vi "getValue.vi"(8 "error in (no error)":errorcluster, 11 "tBSONArray in":refnum<class "tBSONArray.lvclass">) -> (0 "error out":errorcluster, 2 "Value":refnum<class "tBSONElement.lvclass">[](array[class]), 3 "tBSONArray out":refnum<class "tBSONArray.lvclass">)   [LabVIEW 2013, in "BSON.lvlib" / "tBSONArray.lvclass"]
uses:
  tBSONArray.lvclass
  tBSONElement/tBSONElement.lvclass
  tBSONArray.lvclass/tBSONArray.ctl
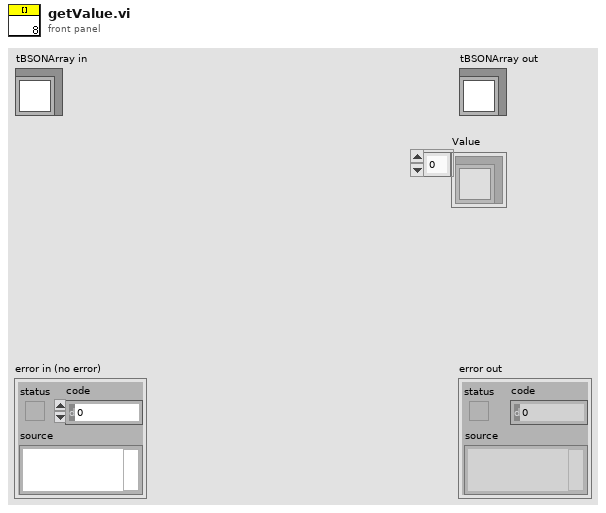
[diagram p1: front panel]
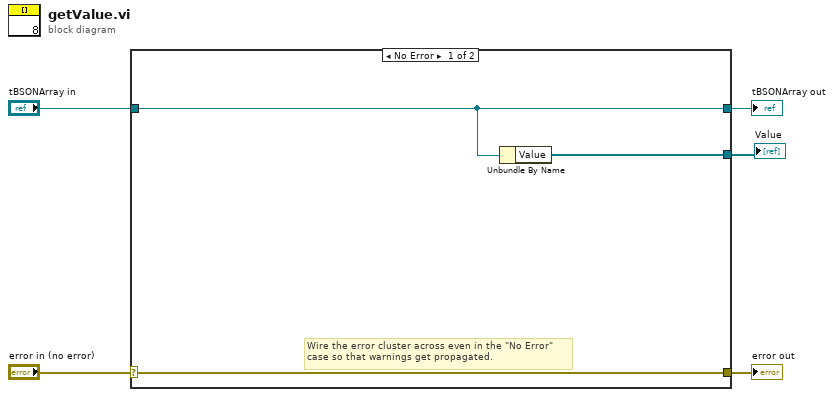
[diagram p0: block diagram]
diagram:
  n1 = case shown="No Error" "error in (no error)" {
    selector: "error in (no error)" -> [w8 w10]
    tunnel: [w8 w10] -> w4
    tunnel: [w7 w9] -> w2
    tunnel: "tBSONArray in" -> [w7 w9]
    tunnel: [w6 _] -> w1
    frame No Error {
      # "Wire the error cluster across even in the \"No Error\"\ncase so that warnings get propagated."
      n2 = Unbundle By Name(w7) -> ("Value"=w6:refnum<class "tBSONElement.lvclass">[])
    }
    frame Error {
    }
  }
  "error out" <- w4
  "tBSONArray out" <- w2
  "Value" <- w1
